vi "TW Call gRPC Scripting.vi"(8 "error in":errorcluster, 10 "gRPC Service Name":string, 11 "proto File Path":path) -> (0 "error out":errorcluster)   [LabVIEW 2021, in "Plugin Generator.lvlib"]
uses:
  Plugin Generator.lvlib
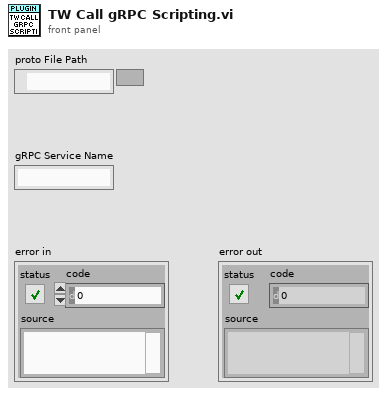
[diagram p1: front panel]
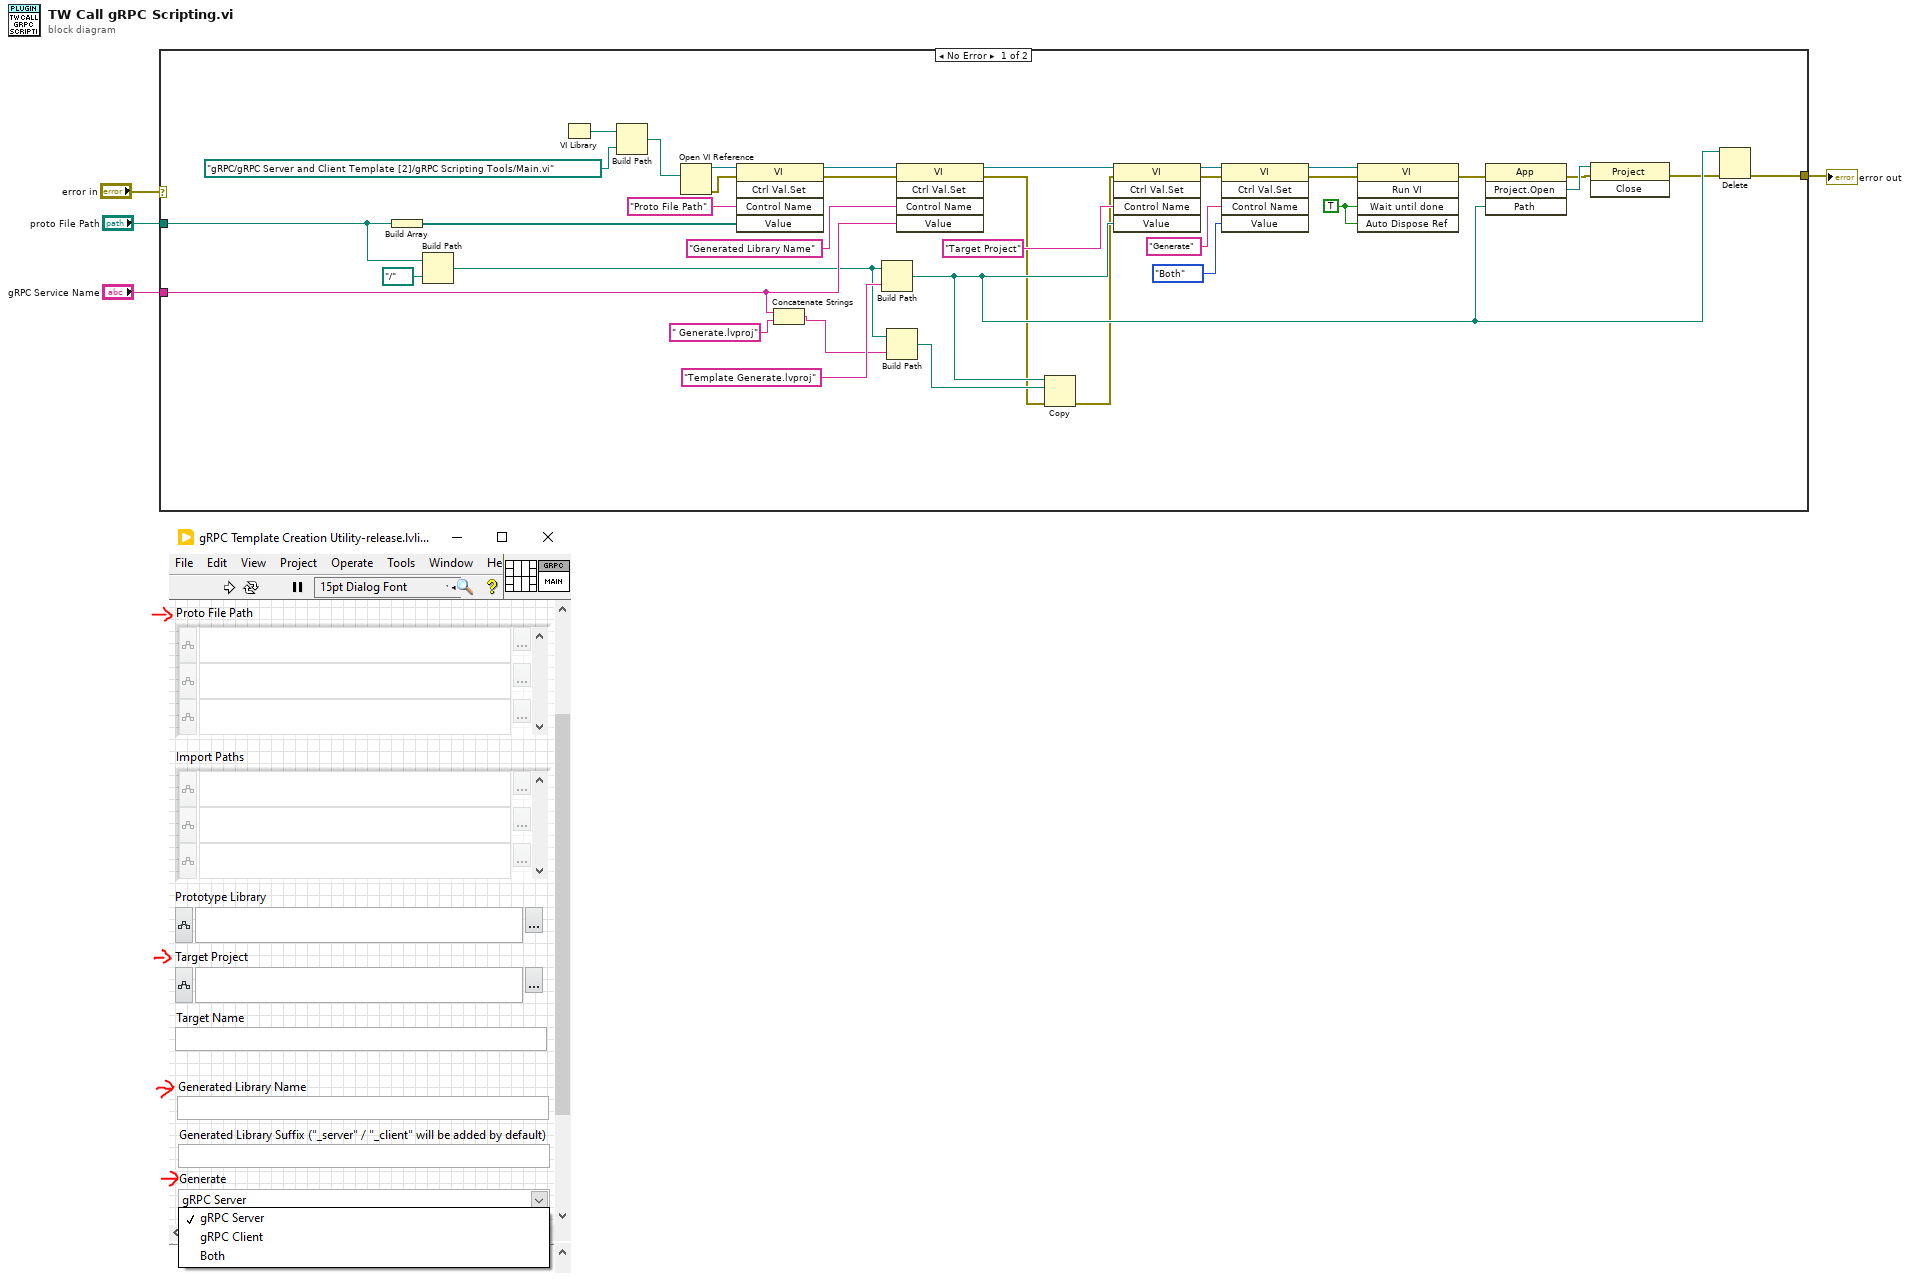
[diagram p0: block diagram]
diagram:
  n1 = case shown="No Error" "error in" {
    selector: "error in" -> [_ w40]
    tunnel: [w9 w40] -> w4
    tunnel: "gRPC Service Name" -> [w16 _]
    tunnel: "proto File Path" -> [w15 _]
    frame No Error {
      w17 = TRUE ("Wait Until Done")
      n2 = Build Array(w15) -> (w22:path[])
      n3 = Build Path(base path=w15, name or relative path=path "../..") -> (appended path=w12:path)
      n4 = VI Library() -> (path=w39:path)
      n5 = Build Path(base path=w39, name or relative path=path "gRPC/gRPC Server and Client Template [2]/gRPC Scripting Tools/Main.vi") -> (appended path=w37:path)
      n6 = Open VI Reference(vi path=w37) -> (vi reference=w24:refnum<vi>, error out=w23:errorcluster)  [unwired: 5 in]
      n7 = invoke class="VI" method="Ctrl Val.Set"(reference=w24, error in=w23, "Control Name"="Proto File Path", "Value"=w22) -> (reference out=w35:refnum<vi>, error out=w34:errorcluster)  [unwired: 1 in, 3 out]
      n8 = Concatenate Strings(w16, " Generate.lvproj" ("string")) -> (w11:string)
      n9 = Build Path(base path=w12, name or relative path="Template Generate.lvproj" ("string")) -> (appended path=w8:path)
      n10 = Build Path(base path=w12, name or relative path=w11) -> (appended path=w10:path)
      n11 = invoke class="VI" method="Ctrl Val.Set"(reference=w35, error in=w34, "Control Name"="Generated Library Name", "Value"=w16) -> (reference out=w32:refnum<vi>, error out=w7:errorcluster)  [unwired: 1 in, 3 out]
      n12 = Copy(8:w7, 10:w10, 11:w8) -> (0:w6:errorcluster)  [unwired: 2 in, 2 out]
      n13 = invoke class="VI" method="Ctrl Val.Set"(reference=w32, error in=w6, "Control Name"="Target Project", "Value"=w8) -> (reference out=w30:refnum<vi>, error out=w29:errorcluster)  [unwired: 1 in, 3 out]
      n14 = invoke class="VI" method="Ctrl Val.Set"(reference=w30, error in=w29, "Control Name"="Generate", "Value"=enum16{"gRPC Server", "gRPC Client", "Both"}."Both" ("Generate")) -> (reference out=w26:refnum<vi>, error out=w25:errorcluster)  [unwired: 1 in, 3 out]
      n15 = invoke class="VI" method="Run VI"(reference=w26, error in=w25, "Wait until done"=w17, "Auto Dispose Ref"=w17) -> (error out=w18:errorcluster)  [unwired: 1 in, 4 out]
      n16 = invoke class="App" method="Project.Open"(error in=w18, "Path"=w8) -> (error out=w19:errorcluster, "Project:Open"=w20:refnum<vi>)  [unwired: 2 in, 2 out]
      n17 = invoke class="Project" method="Close"(reference=w20, error in=w19) -> (error out=w5:errorcluster)  [unwired: 1 in, 2 out]
      n18 = Delete(path (use dialog)=w8, error in=w5) -> (error out=w9:errorcluster)  [unwired: 3 in, 2 out]
    }
    frame Error {
    }
  }
  "error out" <- w4
